vi "test_read_data.vi"() -> ()   [LabVIEW 2011]
panel:
  out "Timer":dbl
  in  "Stop":bool
  out "Cond":dbl
  out "Cap2":dbl
  out "Cap1":dbl
  in  "error in (no error)":errorcluster
  out "error out":errorcluster
  in  "VISA In":refnum<visa-resource-name>
  out "VISA Out":refnum<visa-resource-name>
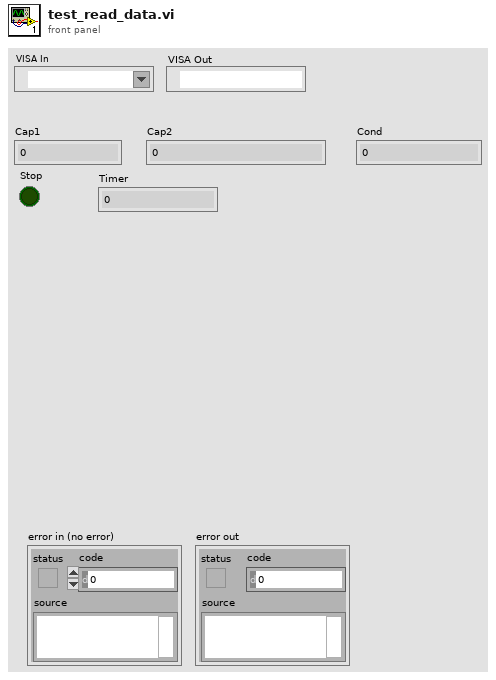
[diagram p1: front panel]
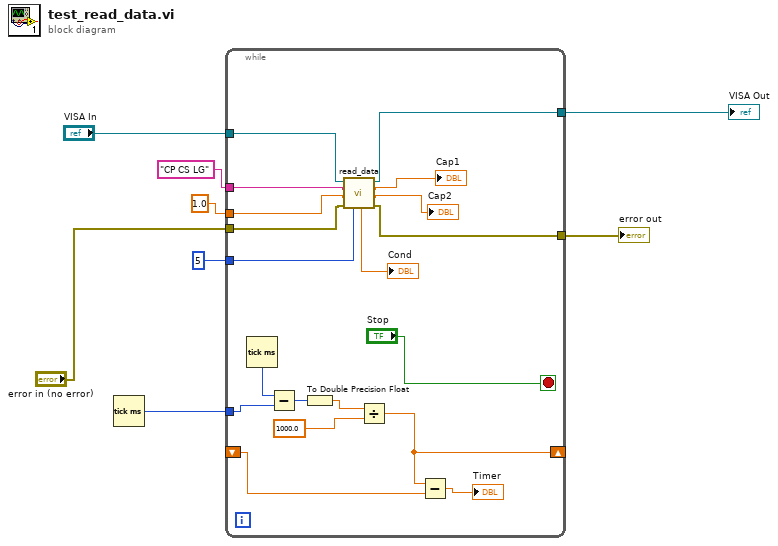
[diagram p0: block diagram]
diagram:
  n1 = Tick Count (ms)() -> (millisecond timer value=w1:u32)
  n2 = while {
    tunnel: "error in (no error)" -> [w24]
    tunnel: "VISA In" -> [w21]
    tunnel: [w20] -> w6
    tunnel: [w17] -> w5
    tunnel: u32 5 ("Samples to Average") -> [w25]
    tunnel: 1.0 ("Read Period") -> [w23]
    tunnel: "CP CS LG" ("Desired Data") -> [w22]
    tunnel: w1 -> [w16]
    shift-right: [w11] -> _
    shift-left: _ -> [w10]
    stop <- "Stop" stop-if-true
    n3 = Tick Count (ms)() -> (millisecond timer value=w15:u32)
    n4 = Subtract(x=w15, y=w16) -> (x-y=w14:u32)
    n5 = To Double Precision Float(number=w14) -> (double precision float=w13:dbl)
    n6 = call "read_data.vi"("Samples to Average"=w25, "error in (no error)"=w24, "Read Period"=w23, "Desired Data"=w22, "VISA In"=w21) -> ("error out"=w17:errorcluster, "Series Cap Avg"=→"Cap2":dbl, "Parallel Cap Avg"=→"Cap1":dbl, "VISA Out"=w20:refnum<visa-resource-name>, "Conductance Avg"=→"Cond":dbl)  [unwired: 2 in]
    n7 = Divide(x=w13, y=1000.0) -> (x/y=w11:dbl)
    n8 = Subtract(x=w11, y=w10) -> (x-y=→"Timer":dbl)
  }
  "VISA Out" <- w6
  "error out" <- w5
